vi "write engine trace msg.vi"(8 "error in (no error)":errorcluster, 9 "Priority":T1(ring)=enum."Debug", 10 "msg":string, 11 "Standard Engine Runtime in":refnum<class "Standard Engine Runtime.lvclass">) -> (0 "error out":errorcluster, 3 "Standard Engine Runtime out":refnum<class "Standard Engine Runtime.lvclass">)   [LabVIEW 2014, in "Standard Engine Runtime.lvclass"]
doc: "Outputs a message to Syslog at the specified priority."
uses:
  Standard Engine Runtime.lvclass
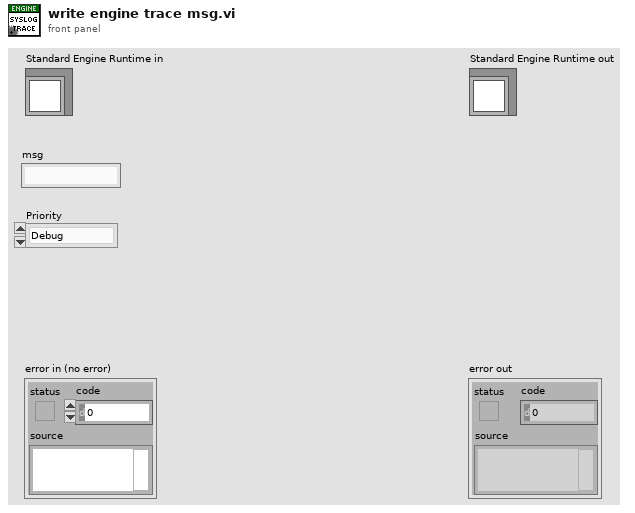
[diagram p1: front panel]
types:
  T1 = enum16{"Emergency", "Alert", "Critical", "Error", "Warning", "Notice", "Informational", "Debug"}
  T2 = enum16{"kern", "user", "mail", "daemon", "auth", "syslog", "lpr", "news", "uucp", "clk", "authpriv", "ftp", "NTP", "log audit", "log alert", "cron", "local0", "local1", "local2", "local3", "local4", "local5", "local6", "local7"}
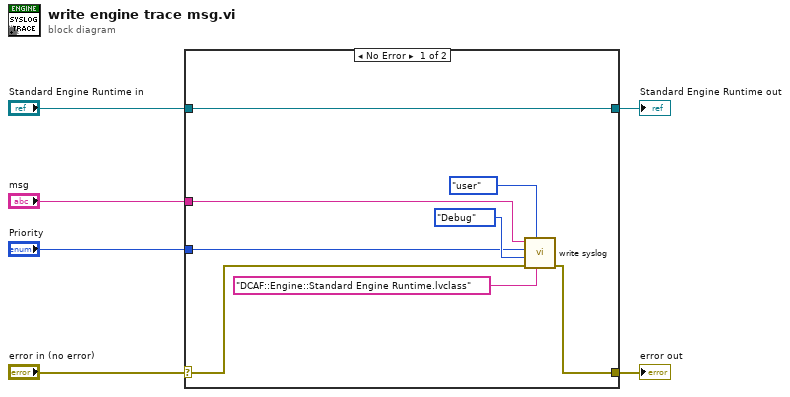
[diagram p0: block diagram]
diagram:
  n1 = case shown="No Error" "error in (no error)" {
    selector: "error in (no error)" -> [w9 w16]
    tunnel: [w8 w16] -> w5
    tunnel: [w14 w15] -> w3
    tunnel: "Standard Engine Runtime in" -> [w14 w15]
    tunnel: "msg" -> [w10 _]
    tunnel: "Priority" -> [w7 _]
    frame No Error {
      n2 = call <vilib>:"write syslog.vi"("prog"="DCAF::Engine::Standard Engine Runtime.lvclass" ("format string"), "Facility"=T2."user", "error in (no error)"=w9, "Minimum level to log"=T1."Debug", "Priority"=w7, "msg"=w10) -> ("error out"=w8:errorcluster)  [unwired: 5 in]
    }
    frame Error {
    }
  }
  "error out" <- w5
  "Standard Engine Runtime out" <- w3
